vi "mean time interval.vi"(6 "init":bool=TRUE, 7 "n":i32=10, 8 "time in":u32) -> (0 "time out":u32, 3 "mean":dbl)   [LabVIEW 2018]
uses:
  <vilib>/Analysis/baseanly.llb/Mean (DBL).vi
  Q - not nan -- integer.vi
  <vilib>/Analysis/NI_AALBase.lvlib
panel:
  out "subarray":u32[](array[numeric])
  out "Array":u32[](array[numeric])
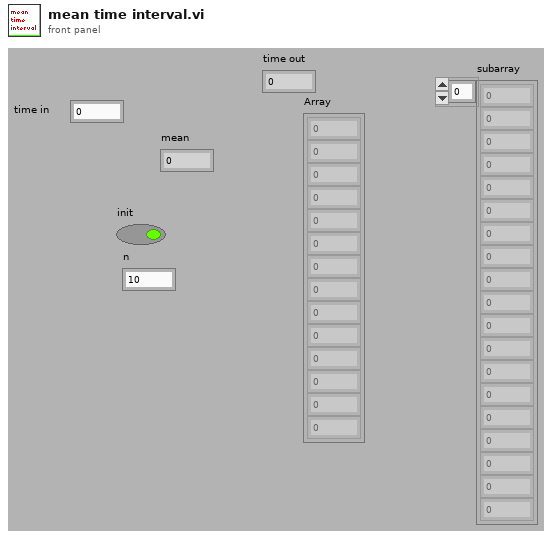
[diagram p1: front panel]
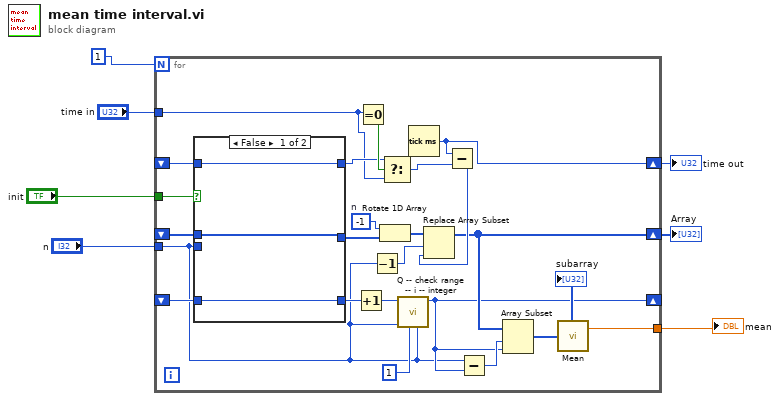
[diagram p0: block diagram]
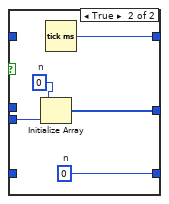
[diagram p2: hidden frame]
diagram:
  n1 = for {
    N: 1 ("n") -> [_]
    tunnel: "init" -> [w30]
    shift-right: [w25] -> w2
    shift-left: _ -> [w26]
    tunnel: "n" -> [w13]
    shift-right: [w19] -> w3
    shift-left: _ -> [w27]
    shift-right: [w14] -> _
    shift-left: _ -> [w22]
    tunnel: [w16] -> w5
    tunnel: "time in" -> [w9]
    w12 = -1  # n
    n2 = case shown="False" w30 {
      tunnel: [w32 w38] -> w10
      tunnel: w13 -> [_ w37]
      tunnel: [w33 w35] -> w28
      tunnel: w27 -> [w33 _]
      tunnel: w26 -> [w32 _]
      tunnel: [w31 w34] -> w23
      tunnel: w22 -> [w31 _]
      frame False {
      }
      frame True {
        w34 = 0  # n
        w36 = u32 0  # n
        n3 = Initialize Array(w36, w37) -> (w35:u32[])
        n4 = Tick Count (ms)() -> (millisecond timer value=w38:u32)
      }
    }
    n5 = Increment(x=w23) -> (x+1=w21:i32)
    n6 = Equal To 0?(x=w9) -> (x = 0?=w11:bool)
    n7 = Decrement(x=w13) -> (x-1=w15:i32)
    n8 = Rotate 1D Array(1:w28, 2:w12) -> (0:w29:u32[])
    n9 = Select(t=w10, s=w11, f=w9) -> (s? t:f=w8:u32)
    n10 = call "Q -- check range -- i -- integer.vi"("upper"=w13, "lower"=1 ("n"), "default"=w13, "number"=w21) -> ("number in range"=w14:i32)  [unwired: 5 in, 2 out]
    n11 = Tick Count (ms)() -> (millisecond timer value=w25:u32)
    n12 = Subtract(x=w25, y=w8) -> (x-y=w24:u32)
    n13 = Replace Array Subset(array=w29, new element=w24, index=w15) -> (w19:u32[])
    n14 = Subtract(x=w13, y=w14) -> (x-y=w18:i32)
    n15 = Array Subset(array=w19, index=w18, length=w14) -> (w17:u32[])
    "subarray" <- w17
    n16 = call-poly <vilib>:"Mean.vi"("X"=w17) -> ("mean"=w16:dbl)  [unwired: 1 out]
  }
  "mean" <- w5
  "Array" <- w3
  "time out" <- w2
